vi "Process_Rect.vi"(11 "XOR Image":T1) -> (1 "Offset Angle From Perpendicular":dbl, 2 "Shortest Dist To Rect Center":dbl, 3 "Processed Image Out":T1)   [LabVIEW 2011]
uses:
  <vilib>/vision/Image Controls.llb/IMAQ Image.ctl
  <vilib>/vision/NI_Vision_Development_Module.lvlib
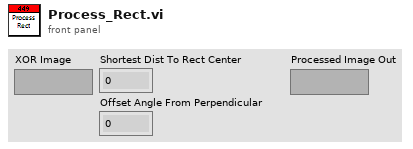
[diagram p1: front panel]
types:
  T1 = typedef "IMAQ Image.ctl" = refnum<image>
  T2 = cluster{"Area":dbl, "Number of Holes":dbl, "Bounding Rect":cluster{"Left":dbl, "Top":dbl, "Right":dbl, "Bottom":dbl}, "Center of Mass":cluster{"X":dbl, "Y":dbl}, "Orientation":dbl, "Dimensions":cluster{"Width":dbl, "Height":dbl}}[]
  T3 = cluster{"Particle Reports (Real-World)  [0]":cluster{"Area":dbl, "Number of Holes":dbl, "Bounding Rect":cluster{"Left":dbl, "Top":dbl, "Right":dbl, "Bottom":dbl}, "Center of Mass":cluster{"X":dbl, "Y":dbl}, "Orientation":dbl, "Dimensions":cluster{"Width":dbl, "Height":dbl}}, "Particle Reports (Real-World)  [1]":cluster{"Area":dbl, "Number of Holes":dbl, "Bounding Rect":cluster{"Left":dbl, "Top":dbl, "Right":dbl, "Bottom":dbl}, "Center of Mass":cluster{"X":dbl, "Y":dbl}, "Orientation":dbl, "Dimensions":cluster{"Width":dbl, "Height":dbl}}, "Particle Reports (Real-World)  [2]":cluster{"Area":dbl, "Number of Holes":dbl, "Bounding Rect":cluster{"Left":dbl, "Top":dbl, "Right":dbl, "Bottom":dbl}, "Center of Mass":cluster{"X":dbl, "Y":dbl}, "Orientation":dbl, "Dimensions":cluster{"Width":dbl, "Height":dbl}}, "Particle Reports (Real-World)  [3]":cluster{"Area":dbl, "Number of Holes":dbl, "Bounding Rect":cluster{"Left":dbl, "Top":dbl, "Right":dbl, "Bottom":dbl}, "Center of Mass":cluster{"X":dbl, "Y":dbl}, "Orientation":dbl, "Dimensions":cluster{"Width":dbl, "Height":dbl}}, "Particle Reports (Real-World)  [4]":cluster{"Area":dbl, "Number of Holes":dbl, "Bounding Rect":cluster{"Left":dbl, "Top":dbl, "Right":dbl, "Bottom":dbl}, "Center of Mass":cluster{"X":dbl, "Y":dbl}, "Orientation":dbl, "Dimensions":cluster{"Width":dbl, "Height":dbl}}, "Particle Reports (Real-World)  [5]":cluster{"Area":dbl, "Number of Holes":dbl, "Bounding Rect":cluster{"Left":dbl, "Top":dbl, "Right":dbl, "Bottom":dbl}, "Center of Mass":cluster{"X":dbl, "Y":dbl}, "Orientation":dbl, "Dimensions":cluster{"Width":dbl, "Height":dbl}}, "Particle Reports (Real-World)  [6]":cluster{"Area":dbl, "Number of Holes":dbl, "Bounding Rect":cluster{"Left":dbl, "Top":dbl, "Right":dbl, "Bottom":dbl}, "Center of Mass":cluster{"X":dbl, "Y":dbl}, "Orientation":dbl, "Dimensions":cluster{"Width":dbl, "Height":dbl}}, "Particle Reports (Real-World)  [7]":cluster{"Area":dbl, "Number of Holes":dbl, "Bounding Rect":cluster{"Left":dbl, "Top":dbl, "Right":dbl, "Bottom":dbl}, "Center of Mass":cluster{"X":dbl, "Y":dbl}, "Orientation":dbl, "Dimensions":cluster{"Width":dbl, "Height":dbl}}, "Particle Reports (Real-World)  [8]":cluster{"Area":dbl, "Number of Holes":dbl, "Bounding Rect":cluster{"Left":dbl, "Top":dbl, "Right":dbl, "Bottom":dbl}, "Center of Mass":cluster{"X":dbl, "Y":dbl}, "Orientation":dbl, "Dimensions":cluster{"Width":dbl, "Height":dbl}}}
  T4 = cluster{"Area":dbl, "Number of Holes":dbl, "Bounding Rect":cluster{"Left":dbl, "Top":dbl, "Right":dbl, "Bottom":dbl}, "Center of Mass":cluster{"X":dbl, "Y":dbl}, "Orientation":dbl, "Dimensions":cluster{"Width":dbl, "Height":dbl}}
  T5 = cluster{"Left":dbl, "Top":dbl, "Right":dbl, "Bottom":dbl}
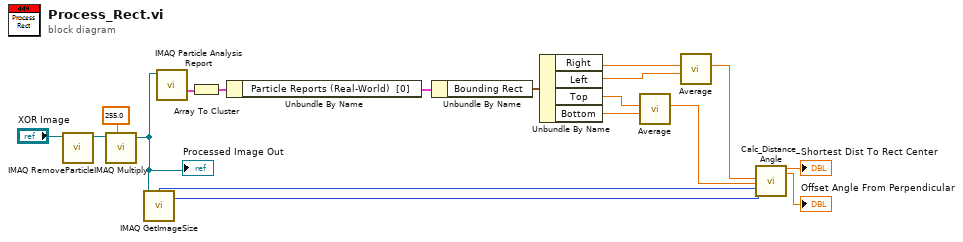
[diagram p0: block diagram]
diagram:
  n1 = call "IMAQ RemoveParticle"("Image Src"="XOR Image") -> ("Image Dst Out"=w11:T1)  [unwired: 9 in, 1 out]
  n2 = call "IMAQ Multiply"("Image Src A"=w11, "Constant"=sgl 255.0) -> ("Image Dst Out"=w12:T1)  [unwired: 5 in, 1 out]
  "Processed Image Out" <- w12
  n3 = call "IMAQ GetImageSize"("Image"=w12) -> ("Y Resolution"=w8:i32, "X Resolution"=w10:i32)  [unwired: 3 in, 1 out]
  n4 = call "IMAQ Particle Analysis Report"("Image"=w12) -> ("Particle Reports (Real-World)"=w16:T2)  [unwired: 5 in, 5 out]
  n5 = Array To Cluster(array=w16) -> (cluster=w15:T3)
  n6 = Unbundle By Name(w15) -> ("Particle Reports (Real-World)  [0]"=w14:T4)
  n7 = Unbundle By Name(w14) -> ("Bounding Rect"=w13:T5)
  n8 = Unbundle By Name(w13) -> ("Right"=w5:dbl, "Left"=w4:dbl, "Top"=w7:dbl, "Bottom"=w6:dbl)
  n9 = call "Average.vi"("B"=w6, "A"=w7) -> ("Avg"=w2:dbl)  [unwired: 9 in]
  n10 = call "Average.vi"("B"=w4, "A"=w5) -> ("Avg"=w3:dbl)  [unwired: 9 in]
  n11 = call "Calc_Distance_Angle.vi"("X Centroid"=w3, "Y Centroid"=w2, "X Resolution"=w10, "Y Resolution"=w8) -> ("Shortest Dist To Rect Cent Inches"=→"Shortest Dist To Rect Center":dbl, "Offset Angle From Perpendicular"=→"Offset Angle From Perpendicular":dbl)  [unwired: 14 in]
